vi "Curve fitting - single curve.vi"() -> ()   [LabVIEW 2016]
uses:
  <vilib>/Analysis/6fits.llb/Curve Fitting Criteria.ctl
  <vilib>/Analysis/NI_AALPro.lvlib
panel:
  out "Portion of curve 2":cluster{dbl[], dbl[]}[](graph)
  out "Fitting Coefficients":dbl[](array[numeric])=[1.9419555129482726e-06, -0.0013073315242499058, 0.0] format="%#_6p"
  in  "Portion of curve":cluster{dbl[], dbl[]}[](graph)=[{array[5855 elements], array[5855 elements]}]
  in  "Section selection":enum32{"Curve section"}(tab)
  in  "length 2":i32=5012
  in  "Starting 2":i32=2389
  out "Data array size":i32=5855
  in  "Section of curve ?":bool
  in  "Fitting type":T1(ring)=enum."Exponential fitting"
  in  "method (least square is default)":T2=2 items=["Least Square", "Least Absolute Residual", "Bisquare"]
  in  "polynomial order":i32=5
  # "For polynomial fitting: Row is the fitting parameter for each curve (from 0th order to nth order).\nFor exponential fitting: Row is the fitting parameter for each curve (amp, damping, offset -- a,b,c for y=a*exp(bx)+c)."
  # "Choose range of each curve"
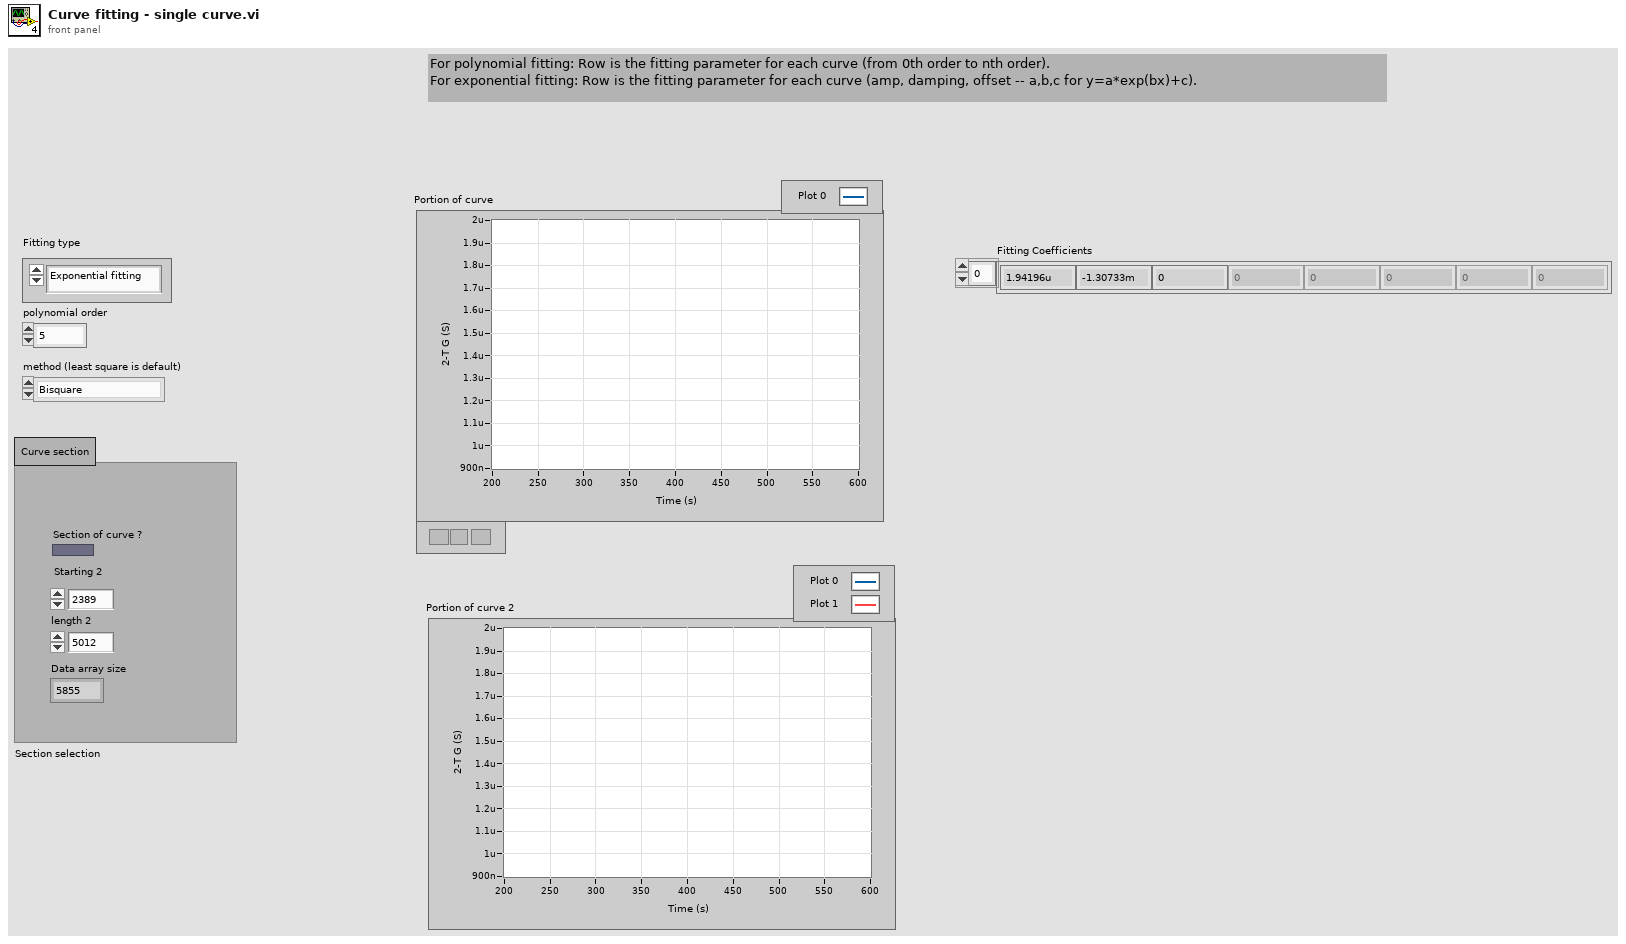
[diagram p1: front panel]
types:
  T1 = enum16{"Polynomial fitting", "Exponential fitting"}
  T2 = typedef "NI_AALPro.lvlib/Curve Fitting Criteria.ctl" = u16
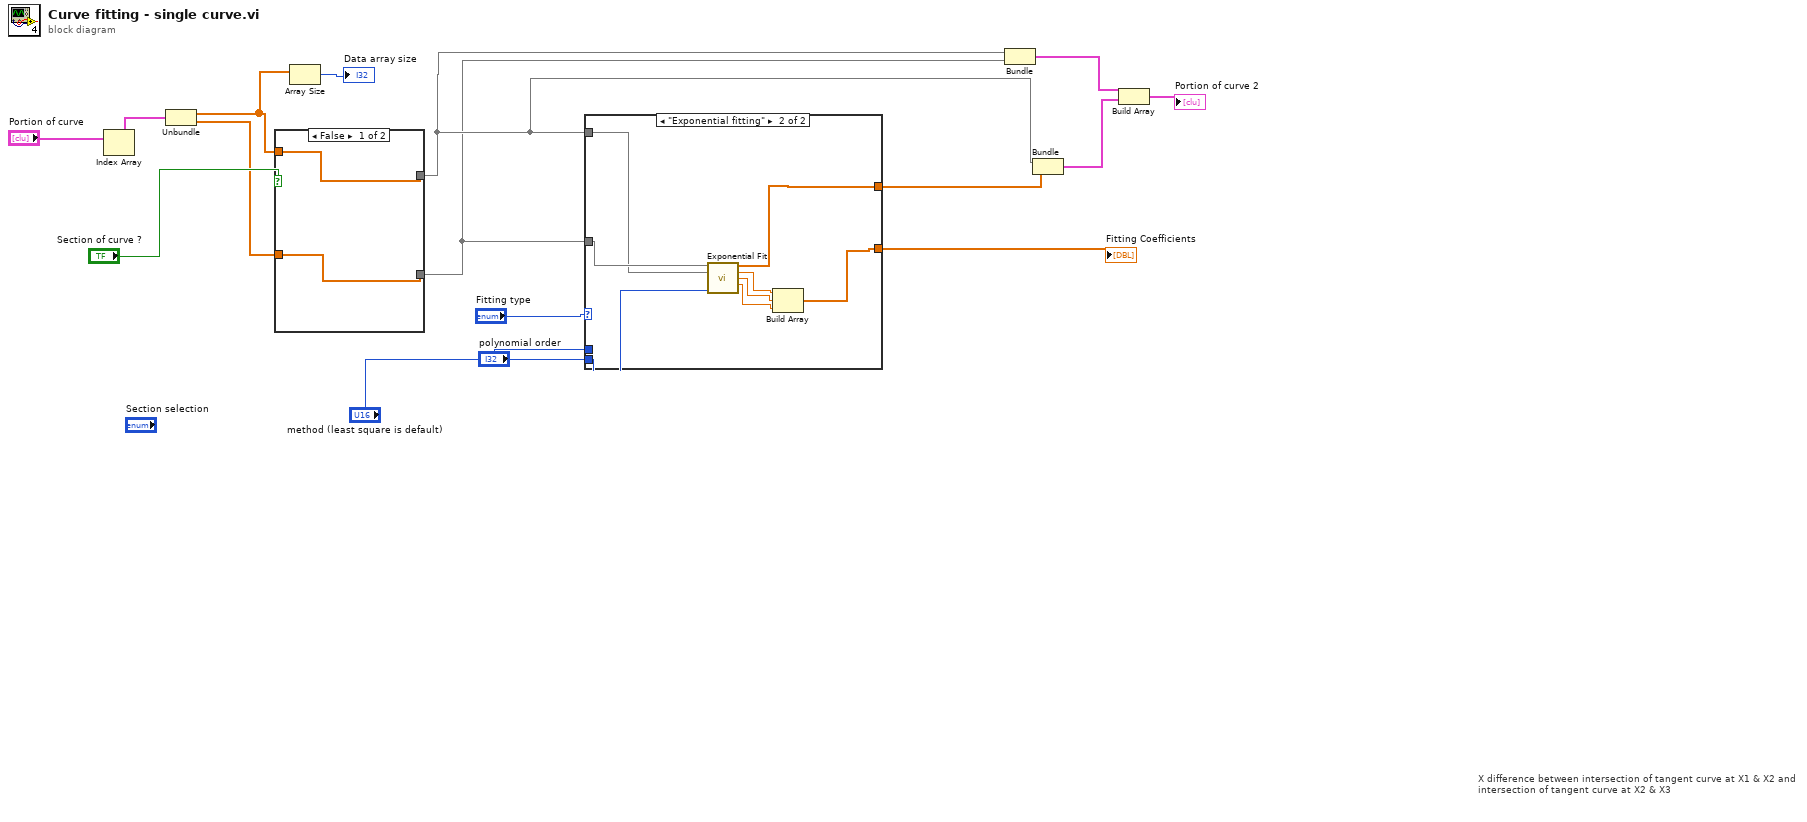
[diagram p0: block diagram]
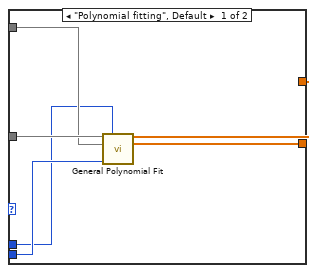
[diagram p2: hidden frame]
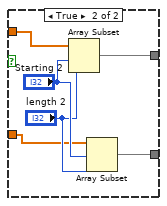
[diagram p3: hidden frame]
diagram:
  # "X difference between intersection of tangent curve at X1 & X2 and intersection of tangent curve at X2 & X3"
  n1 = Index Array(array="Portion of curve") -> (element=w13:cluster{dbl[], dbl[]})  [unwired: 1 in]
  n2 = Unbundle(w13) -> (w3:dbl[], w4:dbl[])
  n3 = case shown="False" "Section of curve ?" {
    tunnel: [w18 w24] -> w2
    tunnel: w4 -> [w17 w19]
    tunnel: [w17 w21] -> w1
    tunnel: w3 -> [w18 w20]
    frame False {
    }
    frame True {
      n4 = Array Subset(array=w20, index="Starting 2", length="length 2") -> (w24:dbl[])
      n5 = Array Subset(array=w19, index="Starting 2", length="length 2") -> (w21:dbl[])
    }
  }
  n6 = Array Size(array=w3) -> (size(s)=→"Data array size":i32)
  n7 = case shown="\"Exponential fitting\"" "Fitting type" {
    tunnel: w1 -> [w30 w38]
    tunnel: w2 -> [w28 w37]
    tunnel: "method (least square is default)" -> [w29 w36]
    tunnel: [w27 w31] -> w10
    tunnel: "polynomial order" -> [w26 _]
    tunnel: [w25 w35] -> w8
    frame "Polynomial fitting", Default {
      n8 = call <vilib>:"General Polynomial Fit.vi"("Y"=w30, "polynomial order"=w26, "X"=w28, "method"=w29) -> ("Best Polynomial Fit"=w25:dbl[], "Polynomial Coefficients"=w27:dbl[])  [unwired: 8 in, 2 out]
    }
    frame "Exponential fitting" {
      n9 = call <vilib>:"Exponential Fit.vi"("Y"=w38, "X"=w37, "method"=w36) -> ("Best Exponential Fit"=w35:dbl[], "amplitude"=w34:dbl, "damping"=w33:dbl, "offset"=w32:dbl)  [unwired: 7 in, 2 out]
      n10 = Build Array(w34, w33, w32) -> (w31:dbl[])
    }
  }
  "Fitting Coefficients" <- w10
  n11 = Bundle(w2, w1) -> (w7:cluster{dbl[], dbl[]})  [unwired: 1 in]
  n12 = Bundle(w2, "Best Exponential Fit"=w8) -> (w6:cluster{dbl[], "Best Exponential Fit":dbl[]})  [unwired: 1 in]
  n13 = Build Array(w7, w6) -> (→"Portion of curve 2":cluster{dbl[], "Best Exponential Fit":dbl[]}[])
